vi "SL TAGS Update From Server-Sync Class Data.vi"(8 "error in (no error)":errorcluster, 10 "Tags to Update":T3[](array[typedef]), 11 "EEISysLink in":refnum<class "EEISysLink.lvclass">) -> (0 "error out":errorcluster, 2 "Updated Tag Values":T1[](array[typedef]), 3 "EEISysLink out":refnum<class "EEISysLink.lvclass">)   [LabVIEW 2017, in "EEISysLink.lvclass"]
doc: "Read the current value of all input tags from the server and update their associated SystemLink class data values. \n\nJames Tillett P.E.\nEndeavor Engineering Inc.\nwww.endeavoreng.com"
uses:
  EEISysLink.lvclass
  Controls/SL Tag.ctl
  <vilib>/Skyline/Tag/Wrapper/Wrapper_class/NI Skyline Tag.lvclass
  Controls/SL Tag Properties.ctl
  Controls/SL Tag Data Type.ctl
  Controls/SL Tag Interpolation Method.ctl
  Controls/SL Tag Unit of Measure.ctl
  Controls/SL Tag Type.ctl
  <vilib>/Skyline/Tag/Shared/typedefs/Tag Cluster.ctl
  <vilib>/Skyline/Tag/Shared/typedefs/DataType.ctl
  Controls/SL Tag Value.ctl
  EEISysLink.lvclass/EEISysLink.ctl
  <vilib>/Skyline/Tag/Shared/NI Skyline Tag.lvlib
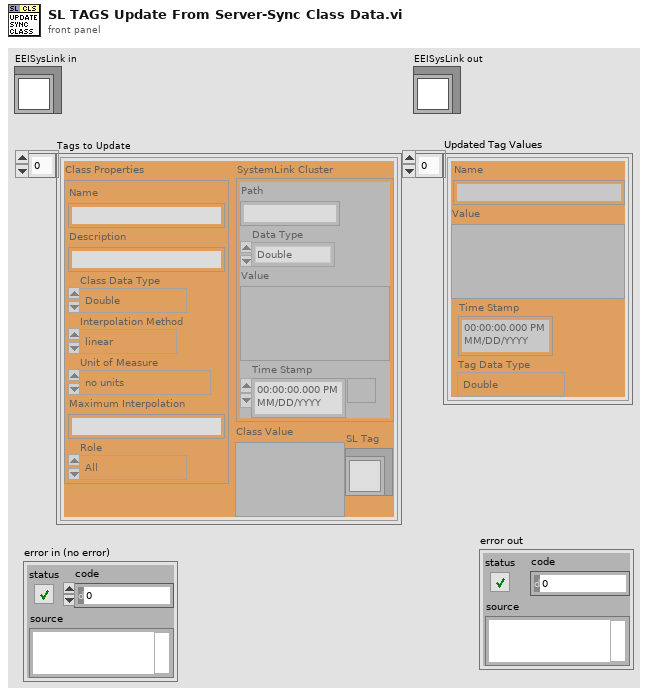
[diagram p1: front panel]
types:
  T1 = typedef "SL Tag Value.ctl" = cluster{"Value":variant, "Time Stamp":timestamp, "Tag Data Type":T2, "Name":string}
  T2 = typedef "EEISysLink.lvclass/SL Tag Data Type.ctl" = enum16{"Double", "Integer", "String", "Boolean", "Waveform"}
  T3 = typedef "EEISysLink.lvclass/SL Tag.ctl" = cluster{"Class Properties":T4, "SL Tag":refnum<class "NI Skyline Tag.lvclass">, "SystemLink Cluster":T8, "Class Value":variant}
  T4 = typedef "EEISysLink.lvclass/SL Tag Properties.ctl" = cluster{"Class Data Type":T2, "Name":string, "Description":string, "Interpolation Method":T5, "Unit of Measure":T6, "Maximum Interpolation":string, "Role":T7}
  T5 = typedef "EEISysLink.lvclass/SL Tag Interpolation Method.ctl" = enum16{"linear", "pilinear", "step"}
  T6 = typedef "EEISysLink.lvclass/SL Tag Unit of Measure.ctl" = enum16{"no units", "Second", "Hour", "Minute", "Day", "Year", "Month", "Week", "Foot", "Yard", "Meter", "Centimeter", "Inch", "Mile", "Nautical Mile", "Miles per Hour", "Meters per second", "Square meter", "Cubic meter", "Cubic centimeter", "Cubic inch", "Liter", "Gallon", "Gallons dry US", "Gallon UK", "Percent", "Revolutions per minute", "Revolution", "Degree angle", "Astronomical Unit", "Atom", "Atomic mass", "Bar", "Byte", "C (speed of light)", "Curie", "Decibel", "Electron Volt", "Ounce", "Knot", "G", "Grade", "Are", "Hectare", "Faraday", "Franklin", "Gilbert", "Erg", "Lambert", "Maxwell", "Gauss", "Electron mass", "Kilogram force", "Pound force", "Rad", "Centiradian", "Sphere", "Mach", "Fluid Ounces", "Fluid Ounces UK", "Fahrenheit", "Celsius", "Kelvin", "Rankine", "Gram", "Kilogram", "Pound", "Short/US Ton", "Long/UK ton", "Metric ton", "Mole", "Pounds per square inch", "Inches water column", "Torr", "Millitorr", "Millimeter mercury", "Inches mercury", "Bar (2)", "Atmosphere", "Pascal", "Watt", "kiloWatt", "Horsepower", "Kilowatt Hour", "British thermal units", "Millions of BTU", "Ampere", "Candela", "Radian", "Steradian", "Bit", "Hertz", "Newton", "Joule", "Coulomb", "Volt", "Farad", "Ohm", "Siemens", "Weber", "Tesla", "Henry", "Lumen", "Lux", "Becqueral", "Gray", "Sievert", "Katal", "Angstrom", "Light Year", "Parsec", "Point", "Pixel", "Dyne", "Kilogram force (2)", "Pound force (2)", "Rem", "Rutherford", "Roentgen"}
  T7 = typedef "EEISysLink.lvclass/SL Tag Type.ctl" = enum16{"All", "Supervisor", "Worker"}
  T8 = typedef "NI Skyline Tag.lvlib/Tag Cluster.ctl" = cluster{"Path":string, "Data Type":T9, "Value":variant, "Time Stamp":timestamp}
  T9 = typedef "NI Skyline Tag.lvlib/DataType.ctl" = enum32{"Double", "Integer", "String"}
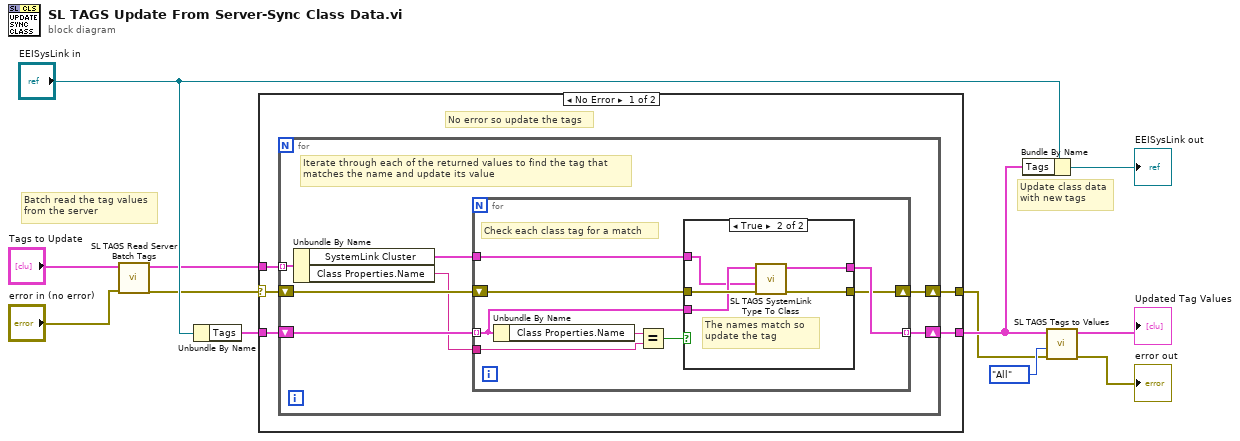
[diagram p0: block diagram]
diagram:
  # "Batch read the tag values\nfrom the server"
  # "Update class data\nwith new tags"
  n1 = call "SL TAGS Read Server Batch Tags.vi"("error in (no error)"="error in (no error)", "Tags In"="Tags to Update") -> ("error out"=w1:errorcluster, "Tags Out"=w2:T3[])  [unwired: 8 in]
  n2 = Unbundle By Name("EEISysLink in") -> ("Tags"=w10:T3[])
  n3 = case shown="No Error" w1 {
    selector: w1 -> [w14 w40]
    tunnel: w10 -> [w17 w41]
    tunnel: w2 -> [w16 _]
    tunnel: [w15 w41] -> w9
    tunnel: [w13 w40] -> w5
    frame No Error {
      # "No error so update the tags"
      n4 = for {
        tunnel: w16 -> [w20] mode=indexing
        shift-right: [w23] -> w15
        shift-left: w17 -> [w24]
        shift-right: [w21] -> w13
        shift-left: w14 -> [w22]
        # "Iterate through each of the returned values to find the tag that\nmatches the name and update its value"
        n5 = Unbundle By Name(w20) -> ("SystemLink Cluster"=w19:T8, "Class Properties.Name"=w18:string)
        n6 = for {
          tunnel: w24 -> [w28] mode=indexing
          tunnel: w18 -> [w31]
          tunnel: w19 -> [w29]
          tunnel: [w27] -> w23 mode=indexing
          shift-right: [w25] -> w21
          shift-left: w22 -> [w26]
          # "Check each class tag for a match"
          n7 = Unbundle By Name(w28) -> ("Class Properties.Name"=w32:string)
          n8 = Equal?(x=w32, y=w31) -> (x = y?=w30:bool)
          n9 = case shown="True" w30 {
            tunnel: w29 -> [_ w37]
            tunnel: w28 -> [w34 w38]
            tunnel: [w34 w36] -> w27
            tunnel: w26 -> [w33 w39]
            tunnel: [w33 w35] -> w25
            frame False {
              # "Names don't match \nso do nothing"
            }
            frame True {
              # "The names match so \nupdate the tag"
              n10 = call "SL TAGS SystemLink Type To Class.vi"("error in (no error)"=w39, "SystemLink Cluster"=w37, "Class Tag In"=w38) -> ("error out"=w35:errorcluster, "Class Tag Out"=w36:T3)  [unwired: 7 in]
            }
          }
        }
      }
    }
    frame Error {
      # "Error on update so don't change tag values"
    }
  }
  n11 = Bundle By Name(cluster="EEISysLink in", "Tags"=w9) -> (→"EEISysLink out":refnum<class "EEISysLink.lvclass">)
  n12 = call "SL TAGS Tags to Values.vi"("error in (no error)"=w5, "Tag Type"=SL_Tag_Type."All", "Tags"=w9) -> ("error out"=→"error out":errorcluster, "Tag Values"=→"Updated Tag Values":T1[])  [unwired: 7 in]
